vi "LNLS Control Decode BPM.vi"(6 "error in (no error)":errorcluster, 8 "command body":string) -> (0 "error out":errorcluster, 3 "BPM Control":u8[](array[numeric]))   [LabVIEW 2011, in "LNLS Control VIs.lvlib"]
uses:
  LNLS Control VIs.lvlib
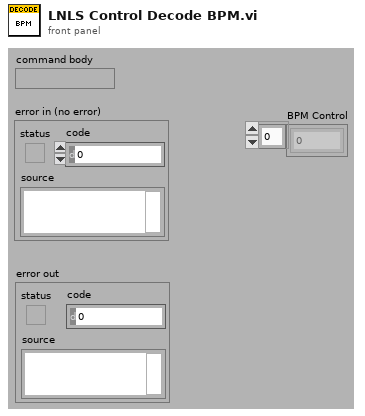
[diagram p1: front panel]
types:
  T1 = enum16{"big-endian, network order", "native, host order", "little-endian"}
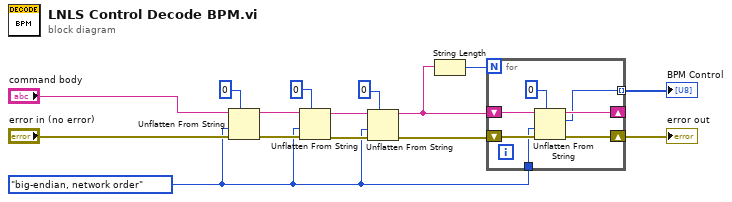
[diagram p0: block diagram]
diagram:
  w3 = T1."big-endian, network order" ("byte order (0:big-endian, network order)")
  n1 = Unflatten From String(type=u8 0 ("priority"), binary string="command body", byte order (0:big-endian, network order)=w3, error in (no error)="error in (no error)") -> (rest of the binary string=w9:string, error out=w13:errorcluster)  [unwired: 1 in, 1 out]
  n2 = Unflatten From String(type=u8 0 ("flag"), binary string=w9, byte order (0:big-endian, network order)=w3, error in (no error)=w13) -> (rest of the binary string=w4:string, error out=w5:errorcluster)  [unwired: 1 in, 1 out]
  n3 = Unflatten From String(type=u16 0 ("number of integrations"), binary string=w4, byte order (0:big-endian, network order)=w3, error in (no error)=w5) -> (rest of the binary string=w2:string, error out=w1:errorcluster)  [unwired: 1 in, 1 out]
  n4 = String Length(string=w2) -> (length=w8:i32)
  n5 = for {
    N: w8 -> [_]
    shift-right: [w17] -> w15
    shift-left: w1 -> [w20]
    shift-right: [w18] -> _
    shift-left: w2 -> [w22]
    tunnel: w3 -> [w19]
    tunnel: [w16] -> w7 mode=indexing
    n6 = Unflatten From String(type=u8 0 ("priority"), binary string=w22, byte order (0:big-endian, network order)=w19, error in (no error)=w20) -> (rest of the binary string=w18:string, value=w16:u8, error out=w17:errorcluster)  [unwired: 1 in]
  }
  "error out" <- w15
  "BPM Control" <- w7
